vi "Main Abstraction Level 0.vi"() -> ()   [LabVIEW 2019]
doc: "This is one of the levels of abstract design along the timeline leading to the goal of a complete measurement application."
panel:
  in  "Record":bool
  in  "Stop":bool
  out "Data":waveform(dbl)[](graph)
  out "Status":string
  in  "Settings":bool
  in  "Start":bool
  in  "Exit":bool
  # "Continuous Measurement Data Logger"
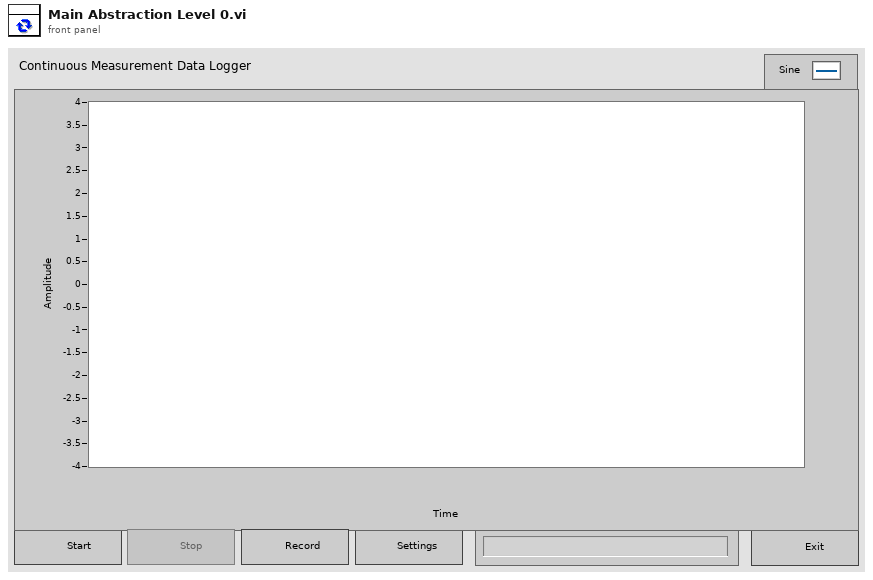
[diagram p1: front panel]
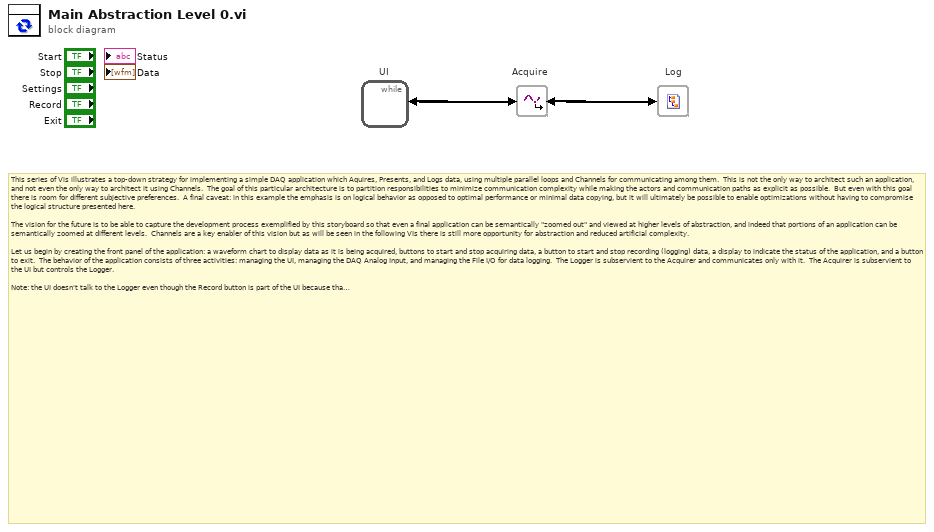
[diagram p0: block diagram]
diagram:
  # "Log"
  # "Acquire"
  # "This series of Vis illustrates a top-down strategy for implementing a simple DAQ application which Aquires, Presents, and Logs data, using multiple parallel loops and Channels for communicating among them.  This is not the only way to architect such an application, and not even the only way to architect it using Channels.  The goal of this particular architecture is to partition responsibilities to minimize communication complexity while making the actors and communication paths as explicit as possible.  But even with this goal there is room for different subjective preferences.  A final caveat: in this example the emphasis is on logical behavior as opposed to optimal performance or minimal data copying, but it will ultimately be possible to enable optimizations without having to compromise the logical structure presented here.\n\nThe vision for the future is to be able to capture the development process exemplified by this storyboard so that even a final application can be semantically \"zoomed out\" and viewed at higher levels of abstraction, and indeed that portions of an application can be semantically zoomed at different levels.  Channels are a key enabler of this vision but as will be seen in the following VIs there is still more opportunity for abstraction and reduced artificial complexity.\n\nLet us begin by creating the front panel of the application: a waveform chart to display data as it is being acquired, buttons to start and stop acquiring data, a button to start and stop recording (logging) data, a display to indicate the status of the application, and a button to exit.  The behavior of the application consists of three activities: managing the UI, managing the DAQ Analog Input, and managing the File I/O for data logging.  The Logger is subservient to the Acquirer and communicates only with it.  The Acquirer is subservient to the UI but controls the Logger.  \n\nNote: the UI doesn't talk to the Logger even though the Record button is part of the UI because that would be redundant (and problematic).  The Acquirer has to know if logging is occurring because it must send the acquired data to the Logger if it is, so it is sufficient (and simpler) for the UI to communicate just with the Acquirer."
  n1 = while "UI" {
    i -> [w2]
    stop <- w1 stop-if-true
    n2 = Greater Than 0?(x=w2) -> (x > 0?=w1:bool)
  }
